vi "CHD_DRIVE_MODULE_ACT.vi"(6 "Pass_Through_Time":dbl=-1.0 format="%33.4f", 9 "Speed Actual":dbl, 10 "Speed Dmd":dbl, 11 "Diff Module TypDef":T1) -> (3 "Wheel Motor Dmd":dbl, 4 "WheelSpeedErr":dbl, 7 "Optimized Speed \nDmd M/S":dbl)   [LabVIEW 2019]
uses:
  <vilib>/Rock Robotics/WPI/ThirdParty/JAS_Junk/TrajLib/Trajectory_Library.lvlib
  CHD_DRIVE_GLOBALS.vi
  <vilib>/Rock Robotics/SystemInterfaces/DIO/FPGA_DIOPWMChannel.ctl
  <vilib>/Rock Robotics/WPI/PWM/WPI_PWMDeadband.ctl
  <vilib>/Rock Robotics/WPI/MotorControl/WPI_MotorControlType.ctl
  <vilib>/Rock Robotics/SystemInterfaces/DIO/FPGA_DIOChannel.ctl
  <vilib>/Rock Robotics/WPI/MotorControl/WPI_MotorControlDeviceRef.ctl
  <vilib>/Rock Robotics/SystemInterfaces/Encoder/FPGA_EncoderIdx.ctl
  <vilib>/Rock Robotics/WPI/Encoder/WPI_EncoderType.ctl
  <vilib>/Rock Robotics/SystemInterfaces/Counter/FPGA_CounterCtrSystemIndex.ctl
  <vilib>/Rock Robotics/WPI/Encoder/WPI_EncoderDevRef.ctl
  CHD_DRIVE_MODULE_TYPDEF.ctl
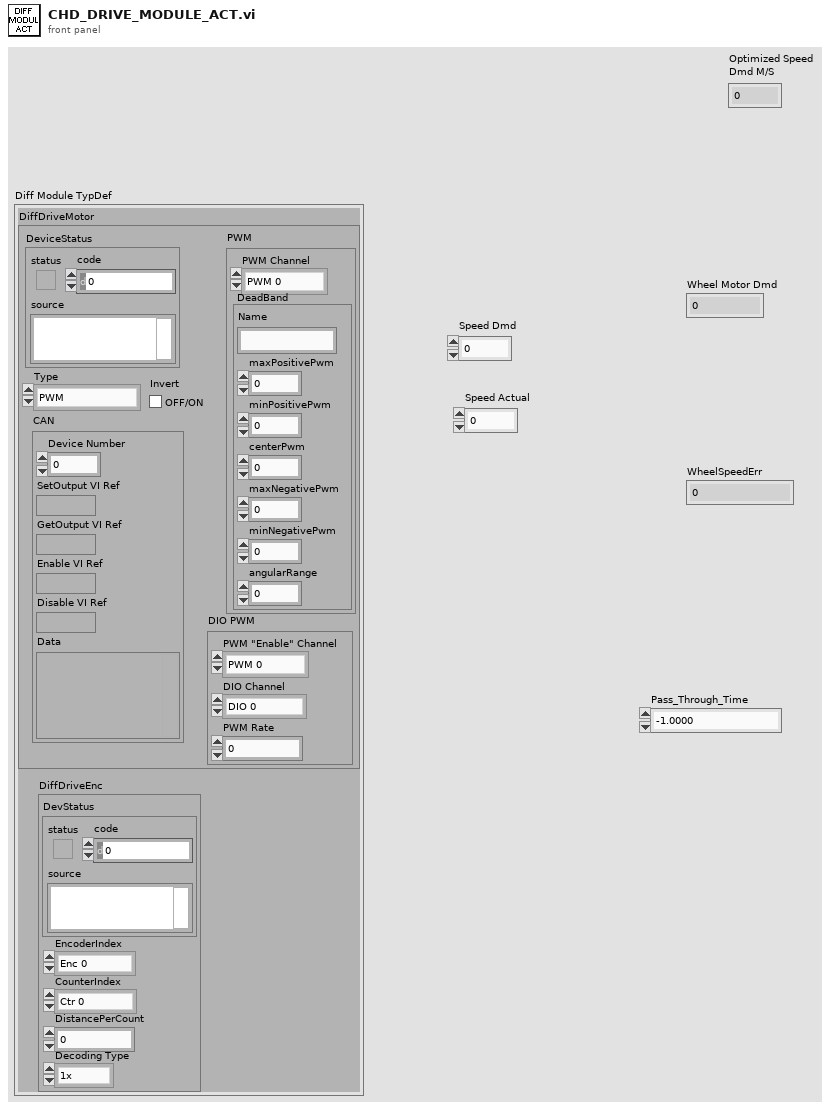
[diagram p1: front panel]
types:
  T1 = typedef "CHD_DRIVE_MODULE_TYPDEF.ctl" = cluster{"DiffDriveMotor":T2, "DiffDriveEnc":T7}
  T2 = typedef "WPI_MotorControlDeviceRef.ctl" = cluster{"DeviceStatus":errorcluster, "Type":T3, "PWM":cluster{"PWM Channel":T4, "DeadBand":T5}, "CAN":cluster{"Device Number":u8, "SetOutput VI Ref":variant, "GetOutput VI Ref":variant, "Enable VI Ref":variant, "Disable VI Ref":variant, "Data":variant}, "Invert":bool, "DIO PWM":cluster{"PWM \"Enable\" Channel":T4, "DIOChannel":T6, "PWM Rate":dbl}}
  T3 = typedef "WPI_MotorControlType.ctl" = enum16{"PWM", "CAN", "DIO PWM"}
  T4 = typedef "FPGA_DIOPWMChannel.ctl" = enum8{"PWM 0", "PWM 1", "PWM 2", "PWM 3", "PWM 4", "PWM 5", "PWM 6", "PWM 7", "PWM 8", "PWM 9", "PWM MXP 0", "PWM MXP 1", "PWM MXP 2", "PWM MXP 3", "PWM MXP 4", "PWM MXP 5", "PWM MXP 6", "PWM MXP 7", "PWM MXP 8", "PWM MXP 9", "Invalid"}
  T5 = typedef "WPI_PWMDeadband.ctl" = cluster{"Name":string, "maxPositivePwm":i32, "minPositivePwm":i32, "centerPwm":i32, "maxNegativePwm":i32, "minNegativePwm":i32, "angularRange":u16}
  T6 = typedef "FPGA_DIOChannel.ctl" = enum8{"DIO 0", "DIO 1", "DIO 2", "DIO 3", "DIO 4", "DIO 5", "DIO 6", "DIO 7", "DIO 8", "DIO 9", "DIO MXP 0", "DIO MXP 1", "DIO MXP 2", "DIO MXP 3", "DIO MXP 4", "DIO MXP 5", "DIO MXP 6", "DIO MXP 7", "DIO MXP 8", "DIO MXP 9", "DIO MXP 10", "DIO MXP 11", "DIO MXP 12", "DIO MXP 13", "DIO MXP 14", "DIO MXP 15", "SPI Port CS1", "SPI Port CS2", "SPI Port CS3", "SPI Port MISO", "SPI Port MOSI", "Invalid"}
  T7 = typedef "WPI_EncoderDevRef.ctl" = cluster{"DevStatus":errorcluster, "EncoderIndex":T8, "CounterIndex":T9, "DistancePerCount":dbl, "Decoding Type":T10}
  T8 = typedef "FPGA_EncoderIdx.ctl" = enum8{"Enc 0", "Enc 1", "Enc 2", "Enc 3", "Enc 4", "Enc 5", "Enc 6", "Enc 7", "Invalid"}
  T9 = typedef "FPGA_CounterCtrSystemIndex.ctl" = enum8{"Ctr 0", "Ctr 1", "Ctr 2", "Ctr 3", "Ctr 4", "Ctr 5", "Ctr 6", "Ctr 7", "Invalid"}
  T10 = typedef "WPI_EncoderType.ctl" = enum16{"1x", "2x", "4x"}
  T11 = typedef "Trajectory_Library.lvlib/PID_ADV_LIMITS.ctl" = cluster{"MaxInput":dbl, "MinInput":dbl, "Continuous":bool, "MaxOutput":dbl, "MinOutput":dbl}
  T12 = typedef "Trajectory_Library.lvlib/PID_ADV_TUNING.ctl" = cluster{"Kf":dbl, "Kp":dbl, "Ki":dbl, "Kd":dbl, "MaximumIntegral":dbl, "MinimumIntegral":dbl, "Filter Derivative":bool, "IntegralZone":dbl}
  T13 = typedef "Trajectory_Library.lvlib/PID_CONTROLLER.ctl" = cluster{"Kp":dbl, "Ki":dbl, "Kd":dbl, "Period":dbl, "Max_Integral":dbl, "Min_Integral":dbl, "Max_Input":dbl, "Min_Input":dbl, "Continuous":bool, "PositionError":dbl, "VelocityError":dbl, "PrevError":dbl, "Total_Integral":dbl, "PositionTolerance":dbl, "VelocityTolerance":dbl, "SetPoint":dbl, "Kf":dbl, "Prev_Deriv":dbl, "Prev_Deriv 2":dbl, "DerivativeFilter":bool, "Min_Output":dbl, "Max_Output":dbl, "Prev_F_P":dbl, "Prev_F_P_2":dbl, "AntiWindupActive":bool, "Measurement":dbl, "IntegralZone":dbl}
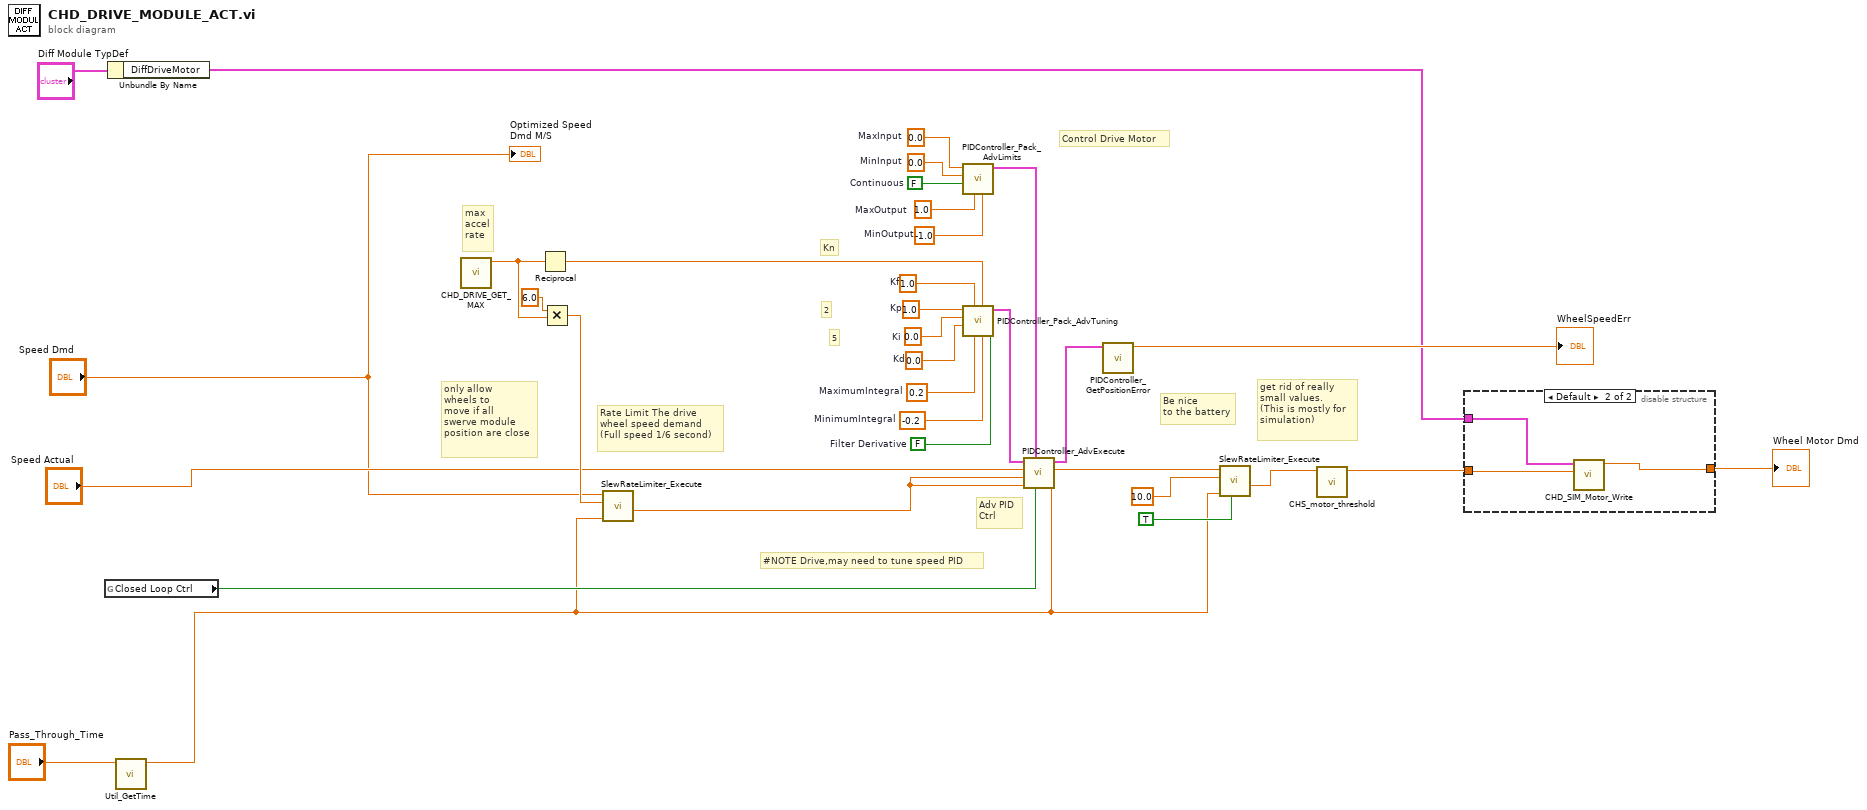
[diagram p0: block diagram]
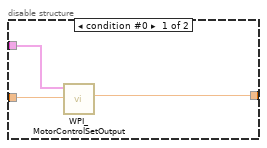
[diagram p2: hidden frame]
diagram:
  w29 = 1.0  # Kp
  w28 = 0.0  # Ki
  w27 = 0.0  # Kd
  w26 = 1.0  # Kf
  w25 = 0.2  # MaximumIntegral
  w24 = -0.2  # MinimumIntegral
  w23 = FALSE  # Filter Derivative
  w21 = 0.0  # MinInput
  w20 = FALSE  # Continuous
  w19 = 1.0  # MaxOutput
  w22 = -1.0  # MinOutput
  w18 = 0.0  # MaxInput
  # "Control Drive Motor"
  # "Be nice\nto the battery"
  # "5"
  # "2"
  # "Kn"
  # "Adv PID\nCtrl"
  # "Rate Limit The drive\nwheel speed demand\n(Full speed 1/6 second)"
  # "only allow\nwheels to \nmove if all \nswerve module \nposition are close"
  # "#NOTE Drive,may need to tune speed PID"
  # "get rid of really\nsmall values.\n(This is mostly for \nsimulation)"
  # "max\naccel\nrate"
  n1 = global read "CHD_DRIVE_GLOBALS.vi" "Closed Loop Ctrl"() -> (w4:bool)
  n2 = Unbundle By Name("Diff Module TypDef") -> ("DiffDriveMotor"=w11:T2)
  n3 = call <vilib>:"Util_GetTime.vi"("Pass_Through_Time"="Pass_Through_Time") -> ("FPGA_Time_Seconds"=w3:dbl)  [unwired: 8 in, 2 out]
  n4 = call "CHD_DRIVE_GET_MAX.vi"() -> ("Max Wheel Vel (Meter/Sec)"=w32:dbl)  [unwired: 11 in]
  n5 = Reciprocal(x=w32) -> (1/x=w15:dbl)
  n6 = Multiply(x=6.0, y=w32) -> (x*y=w31:dbl)
  n7 = call <vilib>:"SlewRateLimiter_Execute.vi"("Time"=w3, "PositiveRate"=w31, "Input"="Speed Dmd") -> ("Output"=w12:dbl)  [unwired: 7 in, 1 out]
  n8 = call <vilib>:"PIDController_Pack_AdvLimits.vi"("MinOutput"=w22, "MaxOutput"=w19, "Continuous"=w20, "MinInput"=w21, "MaxInput"=w18) -> ("Adv PID Limits"=w16:T11)  [unwired: 6 in]
  n9 = call <vilib>:"PIDController_Pack_AdvTuning.vi"("Filter Derivative"=w23, "MinimumIntegral"=w24, "Kn"=w15, "MaximumIntegral"=w25, "Kf"=w26, "Kd"=w27, "Ki"=w28, "Kp"=w29) -> ("Adv PID Tuning"=w17:T12)  [unwired: 3 in]
  n10 = call <vilib>:"PIDController_AdvExecute.vi"("Time"=w3, "Auto"=w4, "Adv PID Limits"=w16, "FF-FeedForward"=w12, "SP-SetPoint"=w12, "PV-Measurement"="Speed Actual", "Adv PID Tuning"=w17) -> ("CO-ControlOutput"=w8:dbl, "out PID_CONTROLLER"=w14:T13)  [unwired: 2 in, 1 out]
  n11 = call <vilib>:"PIDController_GetPositionError.vi"("in PID_CONTROLLER"=w14) -> ("PositionError"=→"WheelSpeedErr":dbl)  [unwired: 10 in]
  n12 = call <vilib>:"SlewRateLimiter_Execute.vi"("Enable"=TRUE, "Time"=w3, "PositiveRate"=10.0, "Input"=w8) -> ("Output"=w7:dbl)  [unwired: 6 in, 1 out]
  n13 = call "CHS_motor_threshold.vi"("motor in"=w7) -> ("motor out"=w10:dbl)  [unwired: 10 in]
  n14 = disable-structure shown="Default" {
    disable-tunnel: w10 -> [w37 w39]
    disable-tunnel: w11 -> [w36 w40]
    disable-tunnel: [w35 w38] -> w9
    frame condition #0 {
      n15 = call <vilib>:"WPI_MotorControlSetOutput.vi"("Output"=w37, "MotorControlDevRef"=w36) -> ("Motor Output"=w35:dbl)  [unwired: 7 in, 2 out]
    }
    frame condition #1 (active) {
      n16 = call "CHD_SIM_Motor_Write.vi"("Motor Demand"=w39, "Motor Device Reference"=w40) -> ("Out Motor Demand"=w38:dbl)  [unwired: 9 in]
    }
  }
  "Wheel Motor Dmd" <- w9
  "Optimized Speed \nDmd M/S" <- "Speed Dmd"
